vi "Circular Buffer (single).vi"(6 "History Length [1024]":i32=1024, 7 "reset":bool, 8 "error in":errorcluster, 11 "XY-data":cluster{"X-array":dbl[], "Y-array":dbl[]} {"Y-array" format="%.2p"; "X-array" format="%.2p"}) -> (0 "error out":errorcluster, 3 "XY-data out":cluster{"X-array":dbl[], "Y-array":dbl[]} {"Y-array" format="%.2p"; "X-array" format="%.2p"})   [LabVIEW 2019, in "xy_utilities.lvlib"]
doc: "Circular Buffer with controllable reset and history length."
uses:
  xy_utilities.lvlib
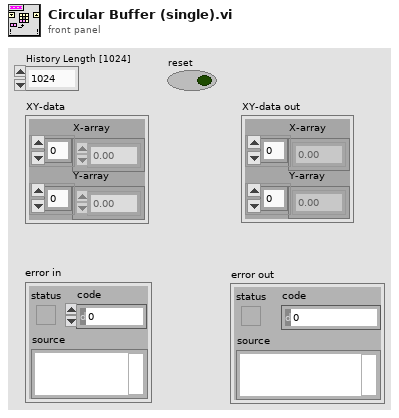
[diagram p1: front panel]
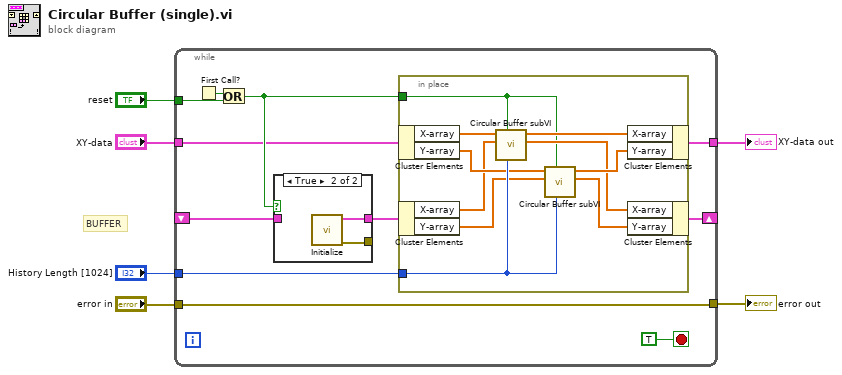
[diagram p0: block diagram]
diagram:
  # "BUFFER"
  n1 = while {
    tunnel: "XY-data" -> [w8]
    tunnel: [w17] -> w3
    tunnel: "error in" -> [w17]
    tunnel: "reset" -> [w15]
    shift-right: [w10] -> _
    shift-left: _ -> [w7]
    tunnel: "History Length [1024]" -> [w13]
    tunnel: [w11] -> w1
    stop <- TRUE stop-if-true
    n2 = First Call?() -> (First Call?: T/F=w16:bool)
    n3 = Or(x=w16, y=w15) -> (x .or. y?=w12:bool)
    n4 = case shown="True" w12 {
      tunnel: w7 -> [w28 _]
      tunnel: [w28 w30] -> w9
      tunnel: [_ w29] -> _
      frame False {
      }
      frame True {
        n5 = call "Initialize.vi"() -> ("error out"=w29:errorcluster, "XY-data out"=w30:cluster{"X-array":dbl[], "Y-array":dbl[]})  [unwired: 10 in]
      }
    }
    n6 = in-place {
      in-place-border: w13 -> [w25]
      in-place-border: w12 -> [w18]
      n7 = in-place-cluster #1(w8) -> ("X-array"=w27:dbl[], "Y-array"=w23:dbl[])
      n8 = in-place-cluster #2(w9) -> ("X-array"=w22:dbl[], "Y-array"=w19:dbl[])
      n9 = call "Circular Buffer subVI.vi"("History Length [1024]"=w25, "Reset"=w18, "Buffer in"=w22, "Array in"=w27) -> ("Buffer out"=w20:dbl[], "Array out"=w26:dbl[])  [unwired: 6 in]
      n10 = call "Circular Buffer subVI.vi"("History Length [1024]"=w25, "Reset"=w18, "Buffer in"=w19, "Array in"=w23) -> ("Buffer out"=w21:dbl[], "Array out"=w24:dbl[])  [unwired: 6 in]
      n11 = in-place-cluster #1("X-array"=w26, "Y-array"=w24) -> (w11:cluster{"X-array":dbl[], "Y-array":dbl[]})
      n12 = in-place-cluster #2("X-array"=w20, "Y-array"=w21) -> (w10:cluster{"X-array":dbl[], "Y-array":dbl[]})
    }
  }
  "XY-data out" <- w1
  "error out" <- w3
